vi "Square Joystick.vi"(11 "In":dbl) -> (3 "Squared Output":dbl)   [LabVIEW 2019]
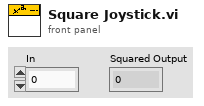
[diagram p1: front panel]
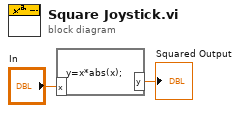
[diagram p0: block diagram]
diagram:
  n1 = formula code="y=x*abs(x);"("x"="In") -> ("y"=→"Squared Output":dbl)
